vi "TestPolishVisionV2.vi"() -> ()   [LabVIEW 2015]
uses:
  <vilib>/vision/Image Controls.llb/IMAQ Image.ctl
  <vilib>/vision/Pattern Matching.llb/IMAQ Curve Parameters.ctl
  <vilib>/vision/Pattern Matching.llb/IMAQ Match Range Setting.ctl
  <vilib>/vision/NI_Vision_Development_Module.lvlib
panel:
  out "Boolean":bool
  in  "error in":errorcluster
  out "Image":T1(plugin-control)
  out "Vison Status":bool
  out "Image Out":T1
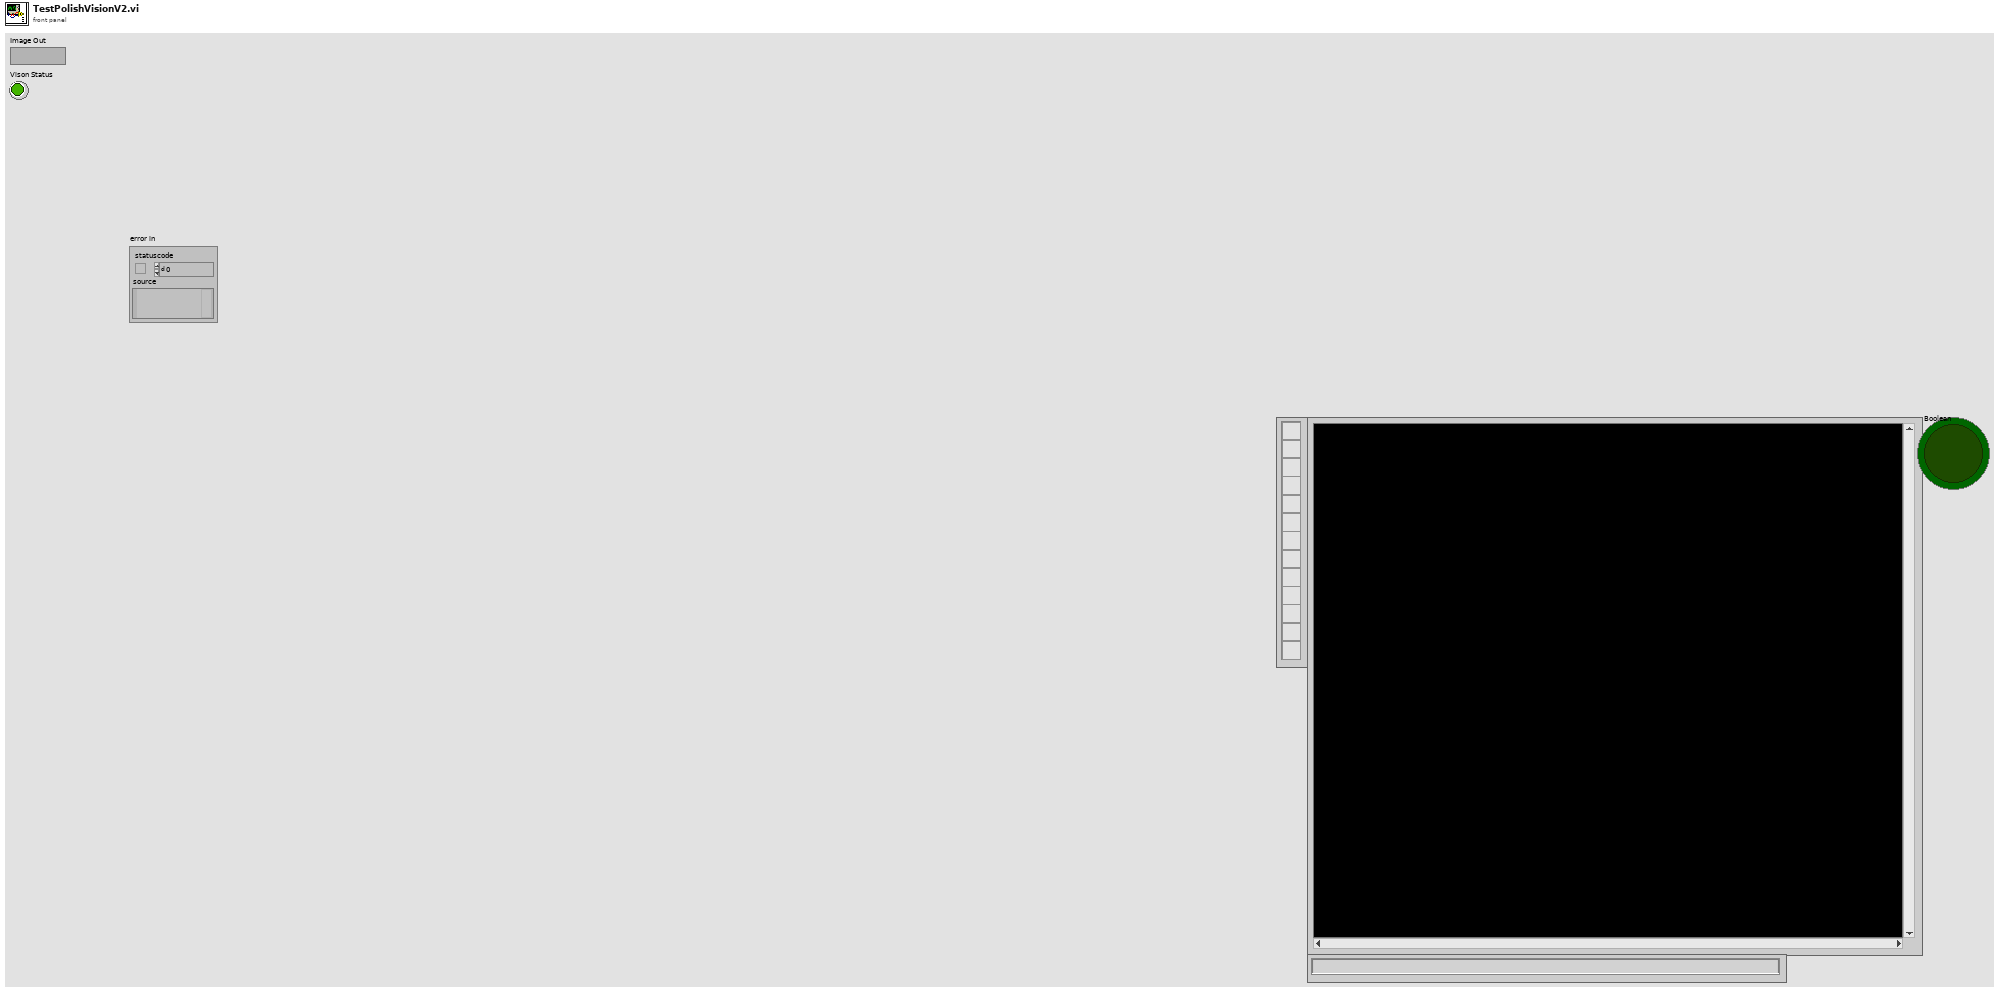
[diagram p1: front panel]
types:
  T1 = typedef "IMAQ Image.ctl" = refnum<image>
  T2 = typedef "Image Type" = u32
  T3 = cluster{"Origin Pixel":cluster{"X":sgl, "Y":sgl}, "X Axis Pixel":cluster{"X":sgl, "Y":sgl}, "Axis Reference":u32}
  T4 = cluster{"Position":cluster{"X":sgl, "Y":sgl}, "Radius":dbl, "Score":dbl}[]
  T5 = cluster{"Circles[0]":cluster{"Position":cluster{"X":sgl, "Y":sgl}, "Radius":dbl, "Score":dbl}, "Circles[1]":cluster{"Position":cluster{"X":sgl, "Y":sgl}, "Radius":dbl, "Score":dbl}, "Circles[2]":cluster{"Position":cluster{"X":sgl, "Y":sgl}, "Radius":dbl, "Score":dbl}, "Circles[3]":cluster{"Position":cluster{"X":sgl, "Y":sgl}, "Radius":dbl, "Score":dbl}, "Circles[4]":cluster{"Position":cluster{"X":sgl, "Y":sgl}, "Radius":dbl, "Score":dbl}, "Circles[5]":cluster{"Position":cluster{"X":sgl, "Y":sgl}, "Radius":dbl, "Score":dbl}, "Circles[6]":cluster{"Position":cluster{"X":sgl, "Y":sgl}, "Radius":dbl, "Score":dbl}, "Circles[7]":cluster{"Position":cluster{"X":sgl, "Y":sgl}, "Radius":dbl, "Score":dbl}, "Circles[8]":cluster{"Position":cluster{"X":sgl, "Y":sgl}, "Radius":dbl, "Score":dbl}}
  T6 = typedef "IMAQ Curve Parameters.ctl" = cluster{"Extraction Mode":u32, "Edge Threshold":i32, "Edge Filter Size":u32, "Min Length":i32, "Row Search Step Size":i32, "Col Search Step Size":i32, "Max Endpoint Gap":i32, "Closed":bool, "Subpixel":bool}
  T7 = typedef "IMAQ Match Range Setting.ctl" = cluster{"Match Constraints":u32, "Min":dbl, "Max":dbl}
  T8 = cluster{"Curve Parameters":T6, "Match Mode":cluster{"Rotation":bool, "Scale":bool, "Occlusion":bool, "Reserved":bool, "Reserved":bool, "Reserved":bool}, "Range Settings":T7[], "Number of Matches":i32, "Minimum Match Score":sgl, "SubPixel Accuracy":bool, "Adv. Geometric Match Options 2":cluster{"Setup Data Item":u16, "Item Value":dbl}[]}
  T9 = cluster{"Global Rectangle":i32[], "Contours":cluster{"ID":enum32{"External", "Internal"}, "Type":u32, "Coordinates":i32[]}[]}
  T10 = typedef "IMAQ GM Match Report.ctl" = cluster{"Position":cluster{"x":sgl, "y":sgl}, "Angle":sgl, "Scale":sgl, "Score":sgl, "Bounding Box":cluster{"x":sgl, "y":sgl}[], "Contrast Reversed":bool, "Occlusion %":sgl, "Template Target Curve Score":sgl, "Target Template Curve Score":sgl, "Correlation Score":sgl}
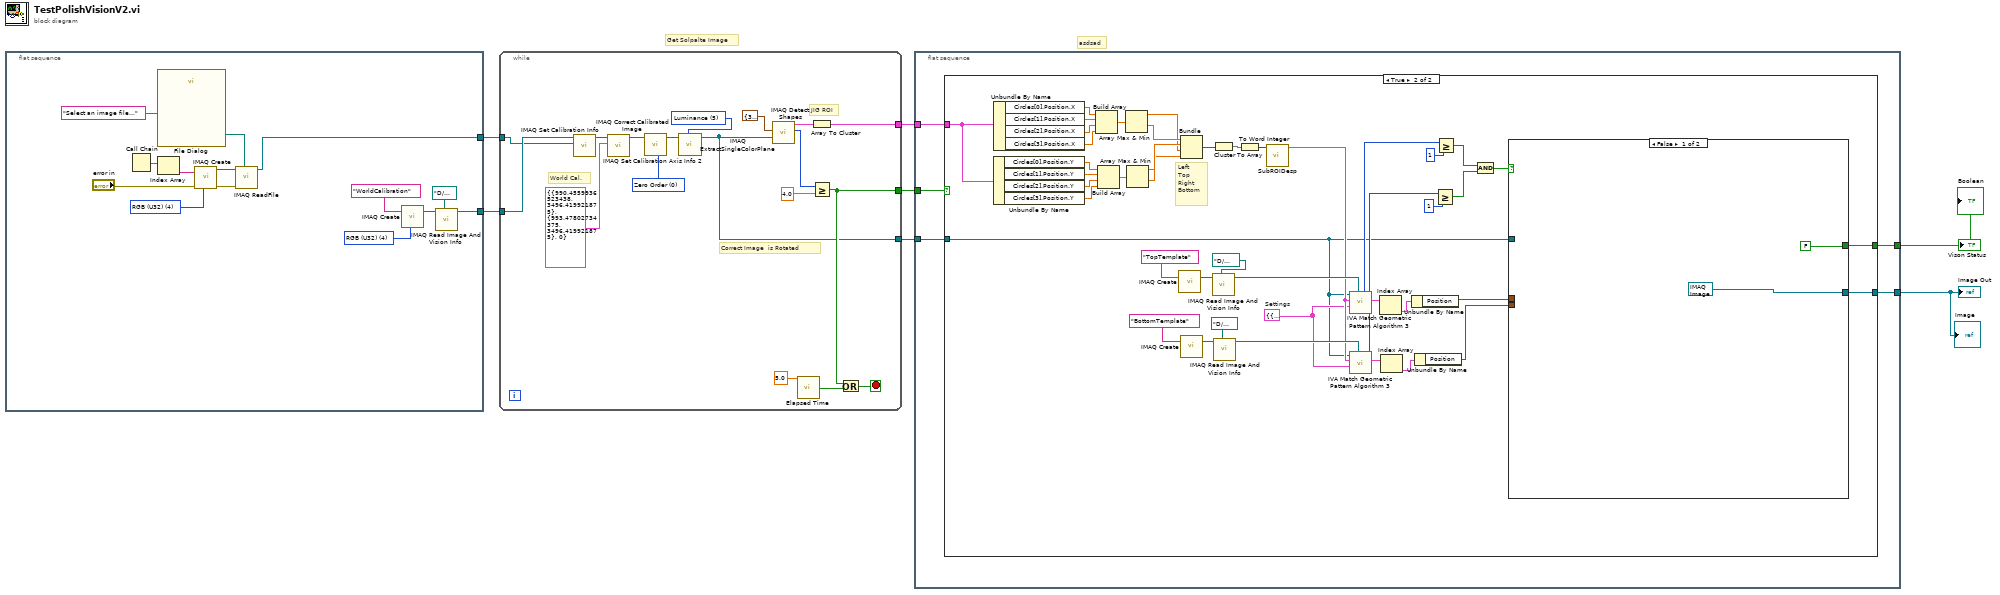
[diagram p0: block diagram]
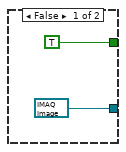
[diagram p2: hidden frame]
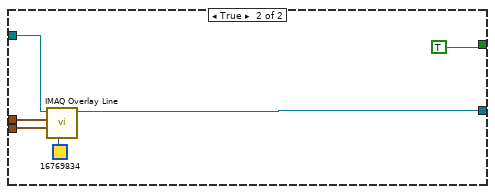
[diagram p3: hidden frame]
diagram:
  # "Get Solpalte Image"
  # "asdsad"
  n1 = flat-sequence {
    tunnel: [w17] -> w7
    tunnel: [w8] -> w1
    frame #0 {
      w9 = T2 4 items=["Grayscale (U8)", "Grayscale (I16)", "Grayscale (SGL)", "Complex (CSG)", "RGB (U32)", "HSL (U32)", "RGB (U64)", "Grayscale (U16)"] ("Image Type")
      w21 = T2 4 items=["Grayscale (U8)", "Grayscale (I16)", "Grayscale (SGL)", "Complex (CSG)", "RGB (U32)", "HSL (U32)", "RGB (U64)", "Grayscale (U16)"] ("Image Type")
      n2 = Call Chain() -> (call chain=w13:string[])
      n3 = Index Array(array=w13) -> (element=w12:string)  [unwired: 1 in]
      n4 = call "File Dialog"("prompt"="Select an image file...") -> ("selected path"=w10:path)  [unwired: 6 in, 8 out]
      n5 = call "IMAQ Create"("Image Name"=w12, "Image Type"=w9, "error in (no error)"="error in") -> ("New Image"=w16:T1, "error out"=w15:errorcluster)  [unwired: 1 in, 1 out]
      n6 = call "IMAQ ReadFile"("File Path"=w10, "error in (no error)"=w15, "Image"=w16) -> ("Image Out"=w8:T1)  [unwired: 2 in, 6 out]
      n7 = call "IMAQ Create"("Image Name"="WorldCalibration", "Image Type"=w21) -> ("New Image"=w19:T1)  [unwired: 2 in, 2 out]
      n8 = call "IMAQ Read Image And Vision Info"("File Path"=path "D:/PolishingRobot/LastEdition/config setting/WorldCalibration.png", "Image"=w19) -> ("Image Out"=w17:T1)  [unwired: 2 in, 7 out]
    }
  }
  n9 = while {
    tunnel: [w29] -> w6
    tunnel: w7 -> [w23]
    tunnel: [w25] -> w5
    tunnel: [w24] -> w4
    tunnel: w1 -> [w22]
    stop <- w26 stop-if-true
    w32 = u32 0 items=["Zero Order", "Bi-Linear", "Quadratic", "Cubic Spline"] ("Interpolation Type")
    w39 = 5 items=["Red", "Green", "Blue", "Hue", "Saturation", "Luminance", "Value", "Intensity"] ("Color Plane")
    # "Correct Image  is Rotated"
    # "World Cal."
    # "JIG ROI"
    n10 = call "IMAQ Set Calibration Info"("Image Dst"=w22, "Image Src"=w23) -> ("Calibrated Image"=w33:T1)  [unwired: 2 in, 7 out]
    n11 = call-poly "IMAQ Set Calibration Axis Info 2"("Calibration Axis Info"=T3 {"Origin Pixel"={"X"=990.456, "Y"=3496.42}, "X Axis Pixel"={"X"=993.478, "Y"=3496.42}, "Axis Reference"=0}, "Calibration Template Image In"=w33) -> ("Calibration Template Image Out"=w31:T1)  [unwired: 1 in, 8 out]
    n12 = call "IMAQ Correct Calibrated Image"("Interpolation Type"=w32, "Image Src"=w31) -> ("Corrected Image"=w30:T1)  [unwired: 5 in, 4 out]
    n13 = call "IMAQ ExtractSingleColorPlane"("Color Plane"=w39, "Image Src"=w30) -> ("Image Dst Out"=w24:T1)  [unwired: 8 in, 1 out]
    n14 = call-poly "IMAQ Detect Shapes"("Circle Descriptor"=cluster{"Min Radius":dbl, "Max Radius":dbl} {"Min Radius"=30.0, "Max Radius"=35.0}, "Image"=w24) -> ("Number of Matches Returned"=w35:i32, "Circles"=w36:T4)  [unwired: 7 in, 1 out]
    n15 = call "Elapsed Time"("Time Target (s)"=5.0) -> ("Time has Elapsed"=w27:bool)  [unwired: 11 in, 7 out]
    n16 = Array To Cluster(array=w36) -> (cluster=w29:T5)
    n17 = Greater Or Equal?(x=w35, y=4.0) -> (x >= y?=w25:bool)
    n18 = Or(x=w25, y=w27) -> (x .or. y?=w26:bool)
  }
  n19 = flat-sequence {
    tunnel: w6 -> [w42]
    tunnel: w5 -> [w44]
    tunnel: w4 -> [w43]
    tunnel: [w41] -> w2
    tunnel: [w40] -> w3
    frame #0 {
      n20 = case shown="True" w44 {
        tunnel: w43 -> [_ w49]
        tunnel: w42 -> [_ w73]
        tunnel: [T1 refnum ("Image Out 2") w48] -> w41
        tunnel: [TRUE w47] -> w40
        frame False {
        }
        frame True {
          w63 = T8 {"Curve Parameters"={"Extraction Mode"=0, "Edge Threshold"=80, "Edge Filter Size"=1, "Min Length"=30, "Row Search Step Size"=10, "Col Search Step Size"=10, "Max Endpoint Gap"=10, "Closed"=FALSE, "Subpixel"=FALSE}, "Match Mode"={"Rotation"=TRUE, "Scale"=FALSE, "Occlusion"=FALSE, "Reserved"=FALSE, "Reserved"=FALSE, "Reserved"=FALSE}, "Range Settings"=[{"Match Constraints"=0, "Min"=-10.0, "Max"=10.0}], "Number of Matches"=1, "Minimum Match Score"=800.0, "SubPixel Accuracy"=FALSE, "Adv. Geometric Match Options 2"=[{"Setup Data Item"=21, "Item Value"=0.0}, {"Setup Data Item"=22, "Item Value"=1.0}]}  # Settings
          # "Left \nTop\nRight \nBottom"
          n21 = Unbundle By Name(w73) -> ("Circles[0].Position.Y"=w78:sgl, "Circles[1].Position.Y"=w77:sgl, "Circles[2].Position.Y"=w76:sgl, "Circles[3].Position.Y"=w75:sgl)
          n22 = Unbundle By Name(w73) -> ("Circles[0].Position.X"=w82:sgl, "Circles[1].Position.X"=w81:sgl, "Circles[2].Position.X"=w80:sgl, "Circles[3].Position.X"=w79:sgl)
          n23 = Build Array(w82, w81, w80, w79) -> (w74:sgl[])
          n24 = Build Array(w78, w77, w76, w75) -> (w72:sgl[])
          n25 = Array Max & Min(array=w74) -> (max value=w69:sgl, min value=w71:sgl)  [unwired: 2 out]
          n26 = Array Max & Min(array=w72) -> (max value=w68:sgl, min value=w70:sgl)  [unwired: 2 out]
          n27 = call "IMAQ Create"("Image Name"="TopTemplate") -> ("New Image"=w89:T1)  [unwired: 3 in, 2 out]
          n28 = call "IMAQ Create"("Image Name"="BottomTemplate") -> ("New Image"=w87:T1)  [unwired: 3 in, 2 out]
          n29 = Bundle(w71, w70, w69, w68) -> (w67:cluster{sgl, sgl, sgl, sgl})  [unwired: 1 in]
          n30 = Cluster To Array(cluster=w67) -> (array=w66:sgl[])
          n31 = call "IMAQ Read Image And Vision Info"("File Path"=path "D:/PolishingRobot/LastEdition/config setting/geomath/Top.png" ("Template File Path"), "Image"=w89) -> ("Image Out"=w84:T1)  [unwired: 2 in, 7 out]
          n32 = call "IMAQ Read Image And Vision Info"("File Path"=path "D:/PolishingRobot/LastEdition/config setting/geomath/bottom.png", "Image"=w87) -> ("Image Out"=w83:T1)  [unwired: 2 in, 7 out]
          n33 = To Word Integer(number=w66) -> (16bit integer=w65:i16[])
          n34 = call "SubROIDesp.vi"("Array"=w65) -> ("output cluster"=w64:T9)  [unwired: 10 in]
          n35 = call <vilib>:"IVA Match Geometric Pattern Algorithm 3.vi"("Template"=w84, "Settings"=w63, "ROI Descriptor"=w64, "Image"=w49) -> ("Matches"=w54:T10[], "Number of Matches"=w62:i32)  [unwired: 1 in, 5 out]
          n36 = call <vilib>:"IVA Match Geometric Pattern Algorithm 3.vi"("Template"=w83, "Settings"=w63, "ROI Descriptor"=w64, "Image"=w49) -> ("Matches"=w56:T10[], "Number of Matches"=w59:i32)  [unwired: 1 in, 5 out]
          n37 = Index Array(array=w54) -> (element=w55:T10)  [unwired: 1 in]
          n38 = Index Array(array=w56) -> (element=w51:T10)  [unwired: 1 in]
          n39 = Unbundle By Name(w55) -> ("Position"=w52:cluster{"x":sgl, "y":sgl})
          n40 = Unbundle By Name(w51) -> ("Position"=w50:cluster{"x":sgl, "y":sgl})
          n41 = Greater Or Equal?(x=w59, y=1) -> (x >= y?=w57:bool)
          n42 = Greater Or Equal?(x=w62, y=1) -> (x >= y?=w58:bool)
          n43 = And(x=w58, y=w57) -> (x .and. y?=w53:bool)
          n44 = case shown="False" w53 {
            tunnel: w52 -> [_ w98]
            tunnel: w50 -> [_ w97]
            tunnel: w49 -> [_ w96]
            tunnel: [T1 refnum ("Image Out 2") w94] -> w48
            tunnel: [FALSE TRUE] -> w47
            frame False {
            }
            frame True {
              n45 = call "IMAQ Overlay Line"("Color"=u32 16769834, "End Point"=w97, "Start Point"=w98, "Image"=w96) -> ("Image Out"=w94:T1)  [unwired: 6 in, 1 out]
            }
          }
        }
      }
    }
  }
  "Image Out" <- w2
  "Vison Status" <- w3
  "Image" <- w2
  "Boolean" <- w3
